vi "ingest_dataflash.vi"(8 "error in":errorcluster, 9 "Target":refnum<class "target.lvclass">, 10 "Source":refnum<class "source.lvclass">, 11 "Nominal Client in":refnum<class "Nominal Client.lvclass">) -> (0 "error out":errorcluster, 1 "datasetRid":string, 2 "datasetFileId":string, 3 "Nominal Client out":refnum<class "Nominal Client.lvclass">)   [LabVIEW 2020, in "Nominal Client.lvclass"]
doc: "Triggers an ingest job, allowing either creating a new dataset or uploading to an existing one. This endpoint is meant to supersede all other ingestion endpoints as their functionality gets migrated to this one."
uses:
  Nominal Client.lvclass
  datasources/target/target.lvclass
  datasources/source/source.lvclass
  Nominal Client.lvclass/Nominal Client.ctl
  datasources/target/target.lvclass/target.ctl
  1ebe6b59-d508-471d-b6f9-c7b5c3253389.vi
  datasources/target/workspace.set.vi
  <vilib>/JDP Science/JSONtext/support/Format JSON Object.vi
  <vilib>/JDP Science/JSONtext/JSON text to Variant.vi
  <vilib>/JDP Science/JSONtext/LVClass Serializer/JSONtext LVClass Serializer.lvclass
  <vilib>/JDP Science/JSONtext/JSONtext.lvlib
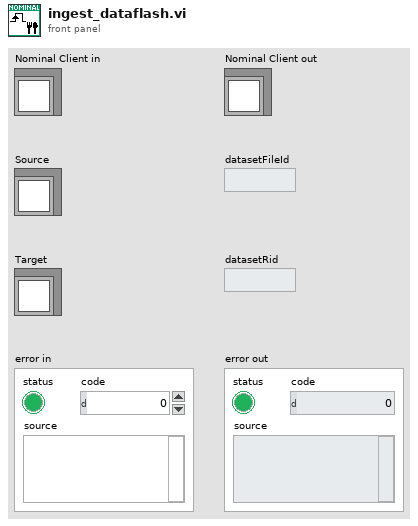
[diagram p1: front panel]
types:
  T1 = cluster{"type":string, "dataset":cluster{"datasetFileId":string, "datasetRid":string}}
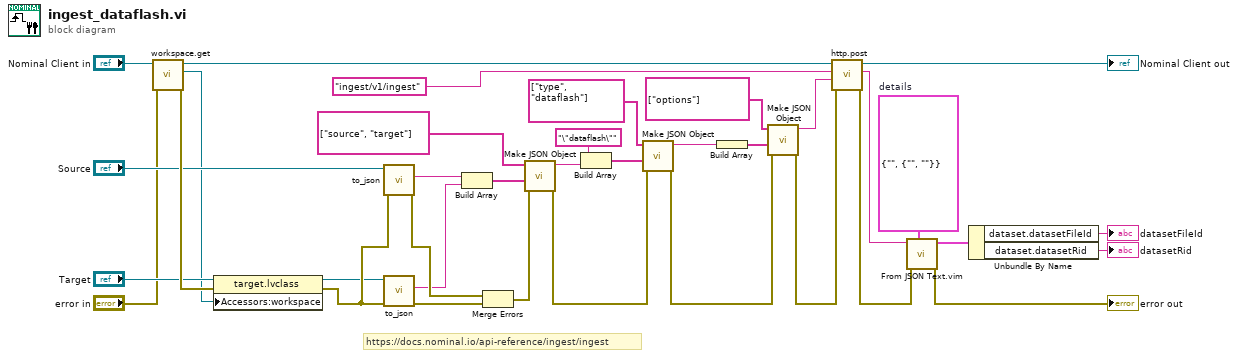
[diagram p0: block diagram]
diagram:
  w13 = T1 {"type"="", "dataset"={"datasetFileId"="", "datasetRid"=""}}  # details
  # "https://docs.nominal.io/api-reference/ingest/ingest"
  n1 = call "workspace.get.vi"("error in"="error in", "Nominal Client in"="Nominal Client in") -> ("error out"=w36:errorcluster, "workspace"=w22:refnum<class "workspace.lvclass">, "Nominal Client out"=w20:refnum<class "Nominal Client.lvclass">)  [unwired: 7 in]
  n2 = property class="target.lvclass"(reference="Target", error in=w36, "Accessors:workspace"=w22) -> (reference out=w23:refnum<class "target.lvclass">, error out=w24:errorcluster)
  n3 = call-dynamic "to_json.vi"("error in"=w24, "source in"="Source") -> ("error out"=w30:errorcluster, "json"=w33:string)  [unwired: 6 in, 2 out]
  n4 = call-dynamic "to_json.vi"("error in"=w24, "target in"=w23) -> ("error out"=w29:errorcluster, "json"=w27:string)  [unwired: 6 in, 2 out]
  n5 = Build Array(w33, w27) -> (w31:string[])
  n6 = Merge Errors(w30, w29) -> (w28:errorcluster)
  n7 = call <vilib>:"Make JSON Object.vi"("error in (no error)"=w28, "JSON Items"=w31, "Item Names"=string[] ["source", "target"] ("Path")) -> ("error out"=w14:errorcluster, "<JSON>"=w15:string)  [unwired: 7 in]
  n8 = Build Array("\"dataflash\"" ("JSON"), w15) -> (w17:string[])
  n9 = call <vilib>:"Make JSON Object.vi"("error in (no error)"=w14, "JSON Items"=w17, "Item Names"=string[] ["type", "dataflash"] ("JSON")) -> ("error out"=w2:errorcluster, "<JSON>"=w5:string)  [unwired: 7 in]
  n10 = Build Array(w5) -> (w6:string[])
  n11 = call <vilib>:"Make JSON Object.vi"("error in (no error)"=w2, "JSON Items"=w6, "Item Names"=string[] ["options"] ("JSON")) -> ("error out"=w1:errorcluster, "<JSON>"=w3:string)  [unwired: 7 in]
  n12 = call "http.post.vi"("error in"=w1, "Request body"=w3, "Path"="ingest/v1/ingest", "Nominal Client in"=w20) -> ("error out"=w12:errorcluster, "Response"=w10:string, "Nominal Client out"=→"Nominal Client out":refnum<class "Nominal Client.lvclass">)  [unwired: 4 in, 1 out]
  n13 = call "From JSON Text.vim"("Data Type and Default Value"=w13, "error in (no error)"=w12, "JSON"=w10) -> ("error out"=→"error out":errorcluster, "Data out"=w9:T1)  [unwired: 7 in]
  n14 = Unbundle By Name(w9) -> ("dataset.datasetFileId"=→"datasetFileId":string, "dataset.datasetRid"=→"datasetRid":string)
